vi "StartRecord.vi"(8 "error in (no error)":errorcluster caption="错误输入（无错误）", 9 "pstRecordParam In":T1, 10 "handle":u64, 11 "strFilePath":u8[](array[numeric])) -> (0 "error out":errorcluster caption="错误输出", 1 "pstRecordParam Out":T1, 2 "handle out":u64, 3 "function return":i32)   [LabVIEW 2013, in "MvCameraControl.lvlib"]
doc: "MV_LV_API int __stdcall SaveImage(MV_SAVE_IMAGE_PARAM* pSaveParam);"
uses:
  MvCameraControl.lvlib
  MvCameraPatch.dll
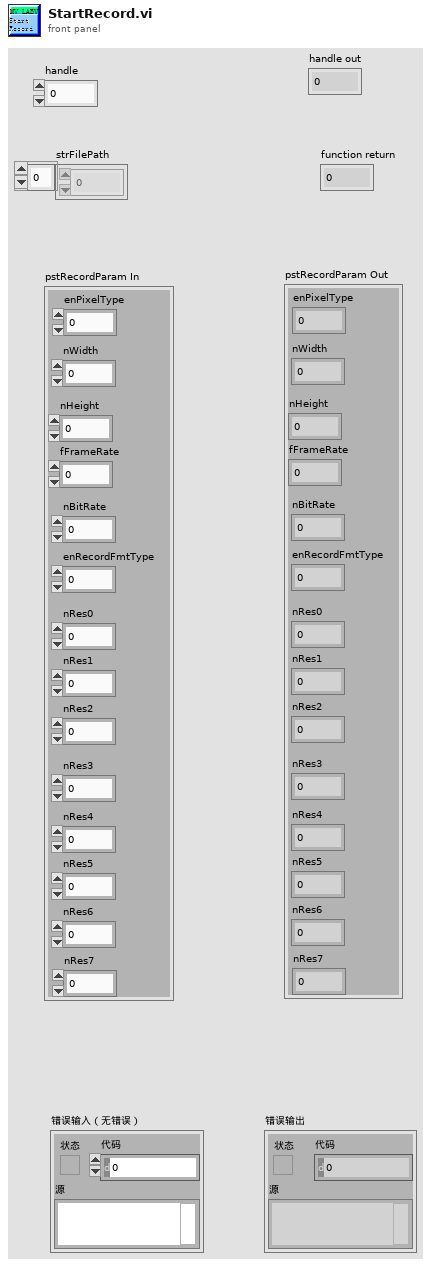
[diagram p1: front panel]
types:
  T1 = cluster{"nWidth":u16, "nHeight":u16, "fFrameRate":sgl, "nBitRate":u32, "enRecordFmtType":i32, "nRes0":u32, "nRes1":u32, "nRes2":u32, "enPixelType":i32, "nRes3":u32, "nRes6":u32, "nRes5":u32, "nRes4":u32, "nRes7":u32}
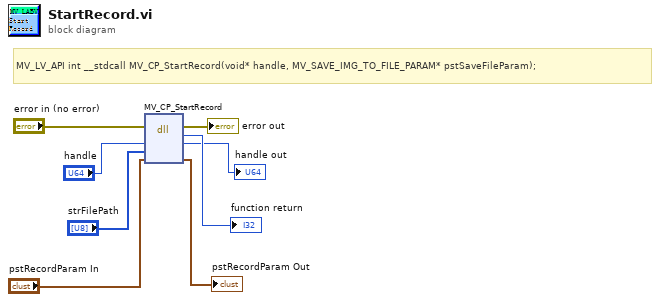
[diagram p0: block diagram]
diagram:
  # "MV_LV_API int __stdcall MV_CP_StartRecord(void* handle, MV_SAVE_IMG_TO_FILE_PARAM* pstSaveFileParam);"
  n1 = dll-call lib="MvCameraPatch.dll" fn="MV_CP_StartRecord"(error in="error in (no error)", "handle"="handle", "strFilePath"="strFilePath", "pstRecordParam"="pstRecordParam In") -> (error out=→"error out":errorcluster, "返回类型"=→"function return":i32, "handle"=→"handle out":u64, "pstRecordParam"=→"pstRecordParam Out":T1)  [unwired: 3 in, 1 out]
